vi "comm wait for bytecount.vi"(7 "loop delay":i32=10, 8 "error in (no error)":errorcluster, 9 "timeout (10000)":u32=10000, 10 "requested byte count":u32, 11 "Comm Handle":u32) -> (0 "error out":errorcluster, 1 "timed out":bool, 2 "actual byte count":u32, 3 "dup Comm Handle":u32)   [LabVIEW 2013, in "lvserial.lvlib"]
doc: "Waits until the requested byte count is in the serial port buffer or the timeout value is reached."
uses:
  lvserial.lvlib
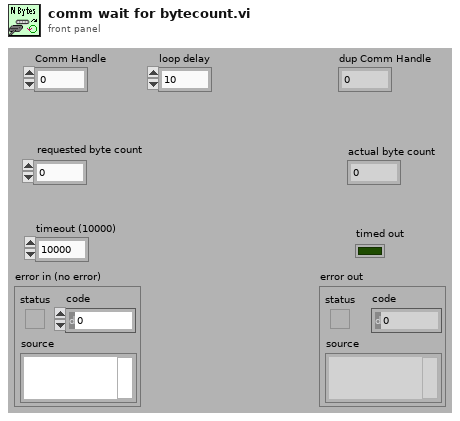
[diagram p1: front panel]
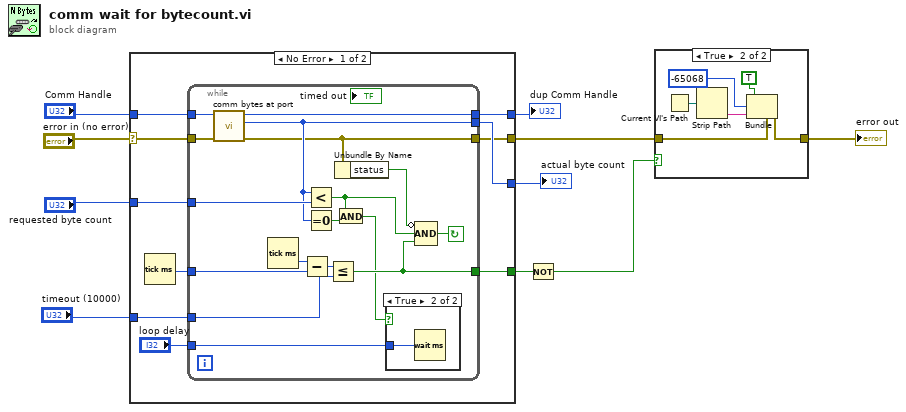
[diagram p0: block diagram]
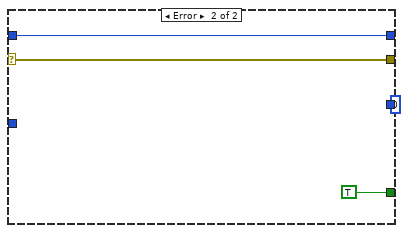
[diagram p3: hidden frame]
diagram:
  n1 = case shown="No Error" "error in (no error)" {
    selector: "error in (no error)" -> [w12 w39]
    tunnel: "Comm Handle" -> [w20 w41]
    tunnel: "requested byte count" -> [w19 _]
    tunnel: "timeout (10000)" -> [w17 _]
    tunnel: [w16 TRUE] -> w8
    tunnel: [w14 w39] -> w9
    tunnel: [w15 u32 0 ("byte count")] -> w3
    tunnel: [w13 w41] -> w2
    frame No Error {
      n2 = Tick Count (ms)() -> (millisecond timer value=w18:u32)
      n3 = while {
        tunnel: "loop delay" -> [w29]
        tunnel: [w22] -> w13
        tunnel: [w23] -> w15
        tunnel: [w30] -> w16
        tunnel: [w21] -> w14
        tunnel: w17 -> [w33]
        tunnel: w18 -> [w35]
        tunnel: w19 -> [w37]
        tunnel: w12 -> [w25]
        tunnel: w20 -> [w24]
        stop <- w31 continue-if-true
        n4 = call "comm bytes at port.vi"("error in (no error)"=w25, "Comm Handle"=w24) -> ("error out"=w21:errorcluster, "bytes at port"=w23:u32, "dup Comm Handle"=w22:u32)  [unwired: 7 out]
        n5 = Tick Count (ms)() -> (millisecond timer value=w36:u32)
        n6 = Subtract(x=w36, y=w35) -> (x-y=w34:u32)
        n7 = Less?(x=w23, y=w37) -> (x < y?=w27:bool)
        n8 = Equal To 0?(x=w23) -> (x = 0?=w28:bool)
        n9 = Less Or Equal?(x=w34, y=w33) -> (x <= y?=w30:bool)
        n10 = Unbundle By Name(w21) -> ("status"=w32:bool)
        n11 = And(x=w27, y=w28) -> (x .and. y?=w26:bool)
        n12 = case shown="True" w26 {
          tunnel: w29 -> [_ w38]
          frame False {
          }
          frame True {
            n13 = Wait (ms)(milliseconds to wait=w38) -> ()  [unwired: 1 out]
          }
        }
        n14 = Compound Arithmetic op=AND(invert w32, w27, w30) -> (w31:bool)
      }
    }
    frame Error {
    }
  }
  "dup Comm Handle" <- w2
  "actual byte count" <- w3
  n15 = Not(x=w8) -> (.not. x?=w10:bool)
  n16 = case shown="True" w10 {
    tunnel: w9 -> [w43 w45]
    tunnel: [w43 w44] -> w1
    frame False {
    }
    frame True {
      n17 = Current VI's Path() -> (path=w47:path)
      n18 = Strip Path(path=w47) -> (name=w48:string)  [unwired: 1 out]
      n19 = Bundle(cluster=w45, "status"=TRUE, "code"=-65068, "source"=w48) -> (w44:errorcluster)
    }
  }
  "error out" <- w1
